vi "Get Topologies.vi"   [LabVIEW 2020, in "SLSC Switch.lvlib"]
doc: "Enumerates the possible SLSC Switch topologies."
uses:
  <vilib>/SLSC_Switch/SLSC Switch.lvlib
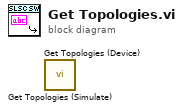
[diagram p0: block diagram]
diagram:
  n1 = call <vilib>:"Get Topologies (Simulate).vi"() -> ()  [unwired: 10 in, 2 out]
  n2 = call <vilib>:"Get Topologies (Device).vi"() -> ()  [unwired: 10 in, 2 out]
